vi "test_MultipleSessionsReserved_CallCloseSessionsWithErrorInput_SessionsClosed.vi"(8 "error in":errorcluster) -> (0 "error out":errorcluster, 2 "result":string, 3 "pass":bool)   [LabVIEW 2020, in "MeasurementServerTests.lvlib"]
uses:
  MeasurementServerTests.lvlib
  Runtime/APIs/Session Management V1/Session Reservation/Session Reservation.lvclass
  Runtime/APIs/Session Management V1/Session Reservation/Connection.ctl
  Runtime/APIs/Session Management V1/Session Reservation/Connection with Session.ctl
  Helpers/Fake Session Factory/Fake Session Factory.lvclass
  e55131ff-ab39-4cad-81ec-f3e0932df67e.vi
  58baf5b5-f2cd-498e-964a-c10dc6bbb2b4.vi
  Runtime/APIs/Session Management V1/Session Reservation/Pin Type.ctl
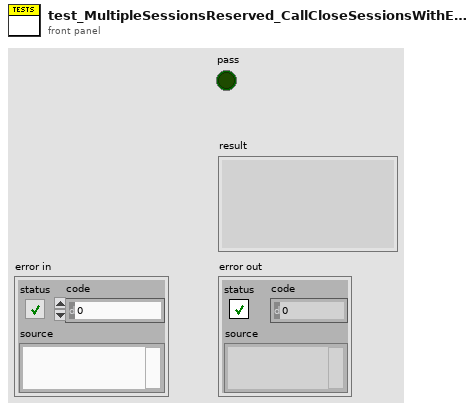
[diagram p1: front panel]
types:
  T1 = typedef "Plug-In SDK Session Management V1 API.lvlib/Session Reservation.lvclass/Pin Type.ctl" = enum16{"DUT and System Pins", "System Pins"}
  T2 = typedef "Plug-In SDK Session Management V1 API.lvlib/Session Reservation.lvclass/Connection with Session.ctl" = cluster{"connection":T3, "session":variant}
  T3 = typedef "Plug-In SDK Session Management V1 API.lvlib/Session Reservation.lvclass/Connection.ctl" = cluster{"pin or relay name":string, "site":i32, "instrument type id":string, "channel":string}
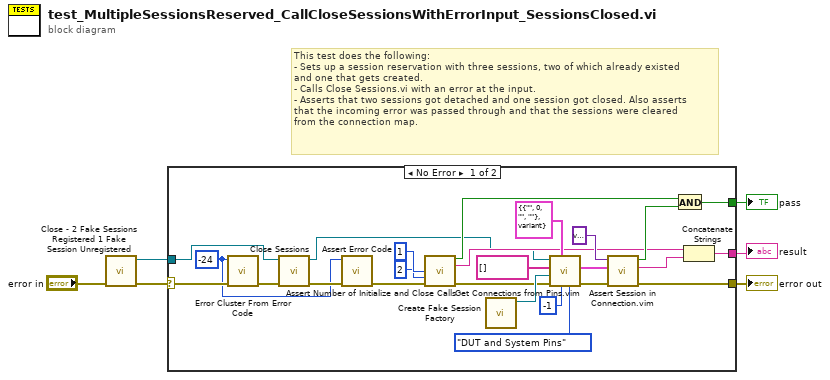
[diagram p0: block diagram]
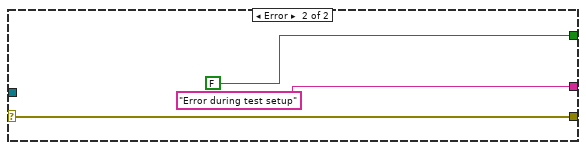
[diagram p2: hidden frame]
diagram:
  # "This test does the following:\n- Sets up a session reservation with three sessions, two of which already existed\nand one that gets created.\n- Calls Close Sessions.vi with an error at the input.\n- Asserts that two sessions got detached and one session got closed. Also asserts\nthat the incoming error was passed through and that the sessions were cleared\nfrom the connection map."
  n1 = call "Close - 2 Fake Sessions Registered 1 Fake Session Unregistered.vi"("error in"="error in") -> ("error out"=w5:errorcluster, "session reservation out"=w4:refnum<class "Session Reservation.lvclass">)  [unwired: 9 in]
  n2 = case shown="No Error" w5 {
    selector: w5 -> [w25 w32]
    tunnel: w4 -> [w30 _]
    tunnel: [w9 w32] -> w3
    tunnel: [w22 FALSE ("pass")] -> w2
    tunnel: [w21 "Error during test setup" ("result")] -> w1
    frame No Error {
      w23 = -24 ("error code (0)")
      n3 = call <vilib>:"Error Cluster From Error Code.vi"("error in (no error)"=w25, "error code (0)"=w23) -> ("error out"=w24:errorcluster)  [unwired: 7 in]
      n4 = call "Close Sessions.vi"("error in"=w24, "session reservation in"=w30) -> ("error out"=w27:errorcluster, "session reservation out"=w8:refnum<class "Session Reservation.lvclass">)  [unwired: 8 in]
      n5 = call "Assert Error Code.vi"("error in"=w27, "expected error code"=w23) -> ("error out"=w26:errorcluster)  [unwired: 7 in, 2 out]
      n6 = call "Assert Number of Initialize and Close Calls.vi"("expected close-close calls"=u32 1, "expected close-detach calls"=u32 2, "error in"=w26) -> ("pass"=w12:bool, "result"=w11:string, "error out"=w14:errorcluster)  [unwired: 10 in]
      n7 = call "Create Fake Session Factory.vi"() -> ("fake session factory out"=w18:refnum<class "Fake Session Factory.lvclass">)  [unwired: 10 in, 1 out]
      n8 = call "Get Connections from Pins.vim"("pin type"=Pin_Type."DUT and System Pins", "site"=-1, "connection type"=T2 {"connection"={"pin or relay name"="", "site"=0, "instrument type id"="", "channel"=""}, "session"=variant}, "error in"=w14, "session factory"=w18, "pin or relay names"=string[] [], "session reservation in"=w8) -> ("error out"=w9:errorcluster, "connections"=w16:T2[])  [unwired: 2 in, 1 out]
      n9 = call "Assert Session in Connection.vim"("actual connections"=w16, "expected session"=variant) -> ("result"=w10:string, "pass"=w13:bool)  [unwired: 8 in]
      n10 = And(x=w12, y=w13) -> (x .and. y?=w22:bool)
      n11 = Concatenate Strings(w11, w10) -> (w21:string)
    }
    frame Error {
    }
  }
  "error out" <- w3
  "pass" <- w2
  "result" <- w1
